vi "16 and 4 pulses TX 1spc.vi"(7 "reset system clock":bool, 8 "referenses":T5={"clock x2"="IO Socket\\Data Clock 2x", "Memory In"="pulse on memory", "Memory In 2"="pulse on memory", "Memory In 3"="pulse on memory", "Memory In 4"="pulse on memory"}, 9 "IQ_run":bool=TRUE, 10 "PDW input Valid":bool, 11 "array PDW":u64[](array[numeric])=[0, 0, 0, 0]) -> (0 "debug mode":T3 {"Cluster"."frequency shift" format="%#_12f"}, 1 "pulse TX status":T6, 2 "output valid":bool, 3 "IQ out":T4, 4 "ready for input":bool)   [LabVIEW 2021]
uses:
  <instrlib>/_niInstr/DSP/v1/Shared/Public/IQ Data.ctl
  pulse_tx_vis/pdw.ctl
  pulse_tx_vis/CTL/mode_type.ctl
  <instrlib>/_niInstr/Basic Elements/v1/FPGA/Private/Count Up U64.vi
  <instrlib>/_niInstr/Basic Elements/v1/FPGA/Private/Count Up U32.vi
  <instrlib>/_niInstr/Basic Elements/v1/FPGA/niInstr Basic Elements v1 FPGA.lvlib
  <instrlib>/_niInstr/DSP/v1/Shared/niInstr DSP v1 Shared.lvlib
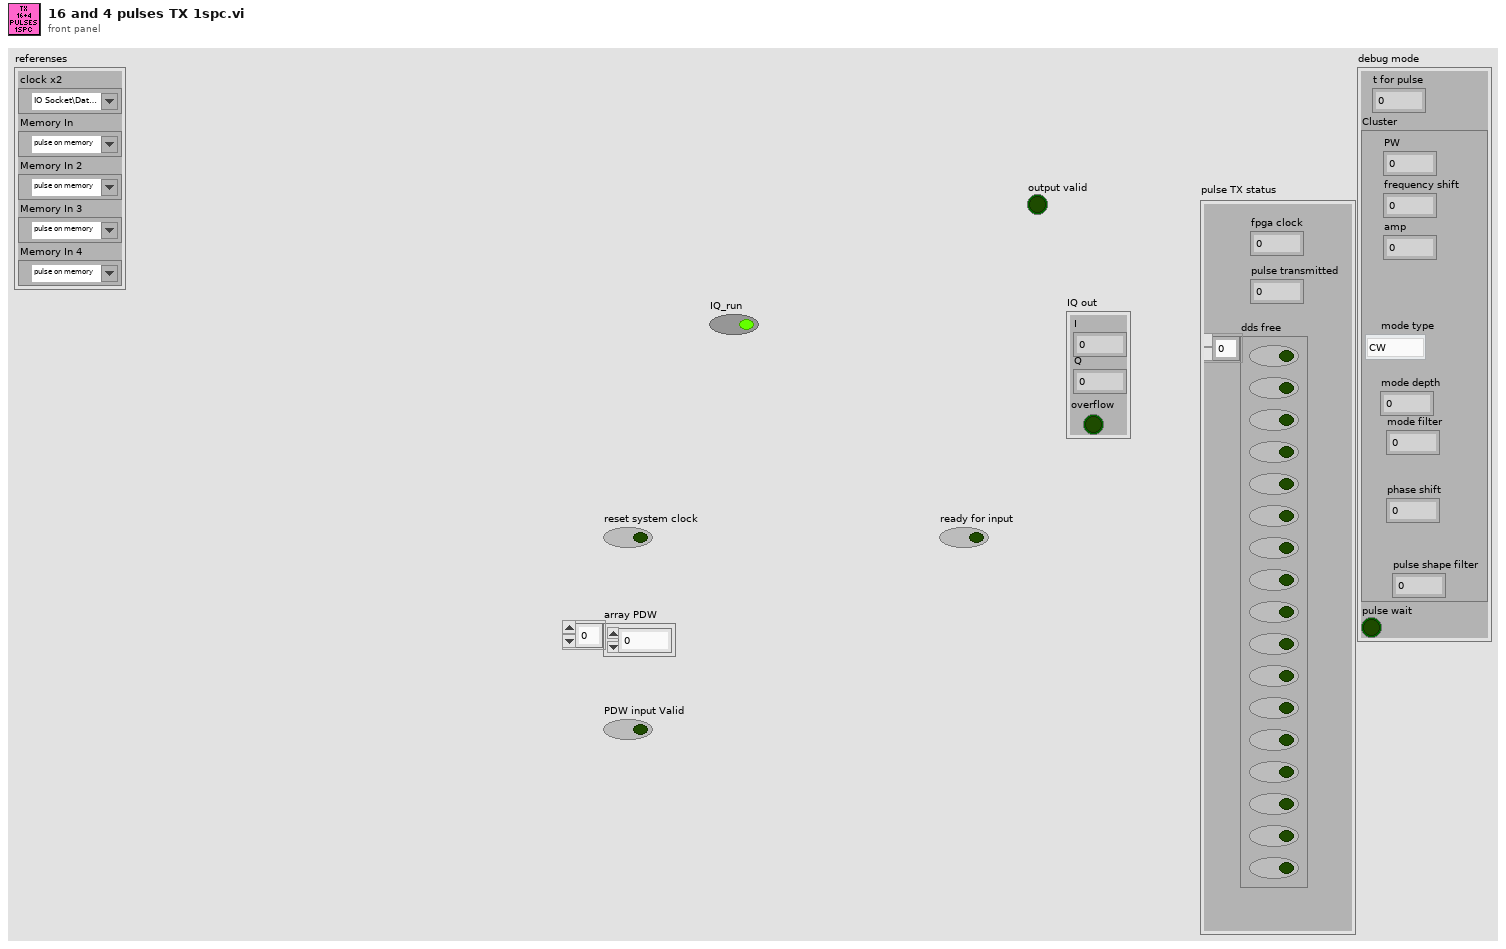
[diagram p1: front panel]
types:
  T1 = typedef "pdw.ctl" = cluster{"PW":u32, "frequency shift":fxp<+/-,48,0>, "amp":fxp<+/-,18,1>, "mode type":T2, "mode depth":u32, "mode filter":u8, "phase shift":fxp<+/-,16,1>, "pulse shape filter":u8}
  T2 = typedef "mode_type.ctl" = enum8{"CW", "from memory 1", "NC - cw", "LFM", "BPSK", "QPSK"}
  T3 = cluster{"t for pulse":u64, "Cluster":T1, "pulse wait":bool}
  T4 = typedef "niInstr DSP v1 Shared.lvlib/IQ Data.ctl" = cluster{"I":fxp<+/-,18,1>, "Q":fxp<+/-,18,1>, "overflow":bool}
  T5 = cluster{"clock x2":refnum<k21>, "Memory In":refnum<k21>, "Memory In 2":refnum<k21>, "Memory In 3":refnum<k21>, "Memory In 4":refnum<k21>}
  T6 = cluster{"fpga clock":u64, "pulse transmitted":u32, "dds free":bool[]}
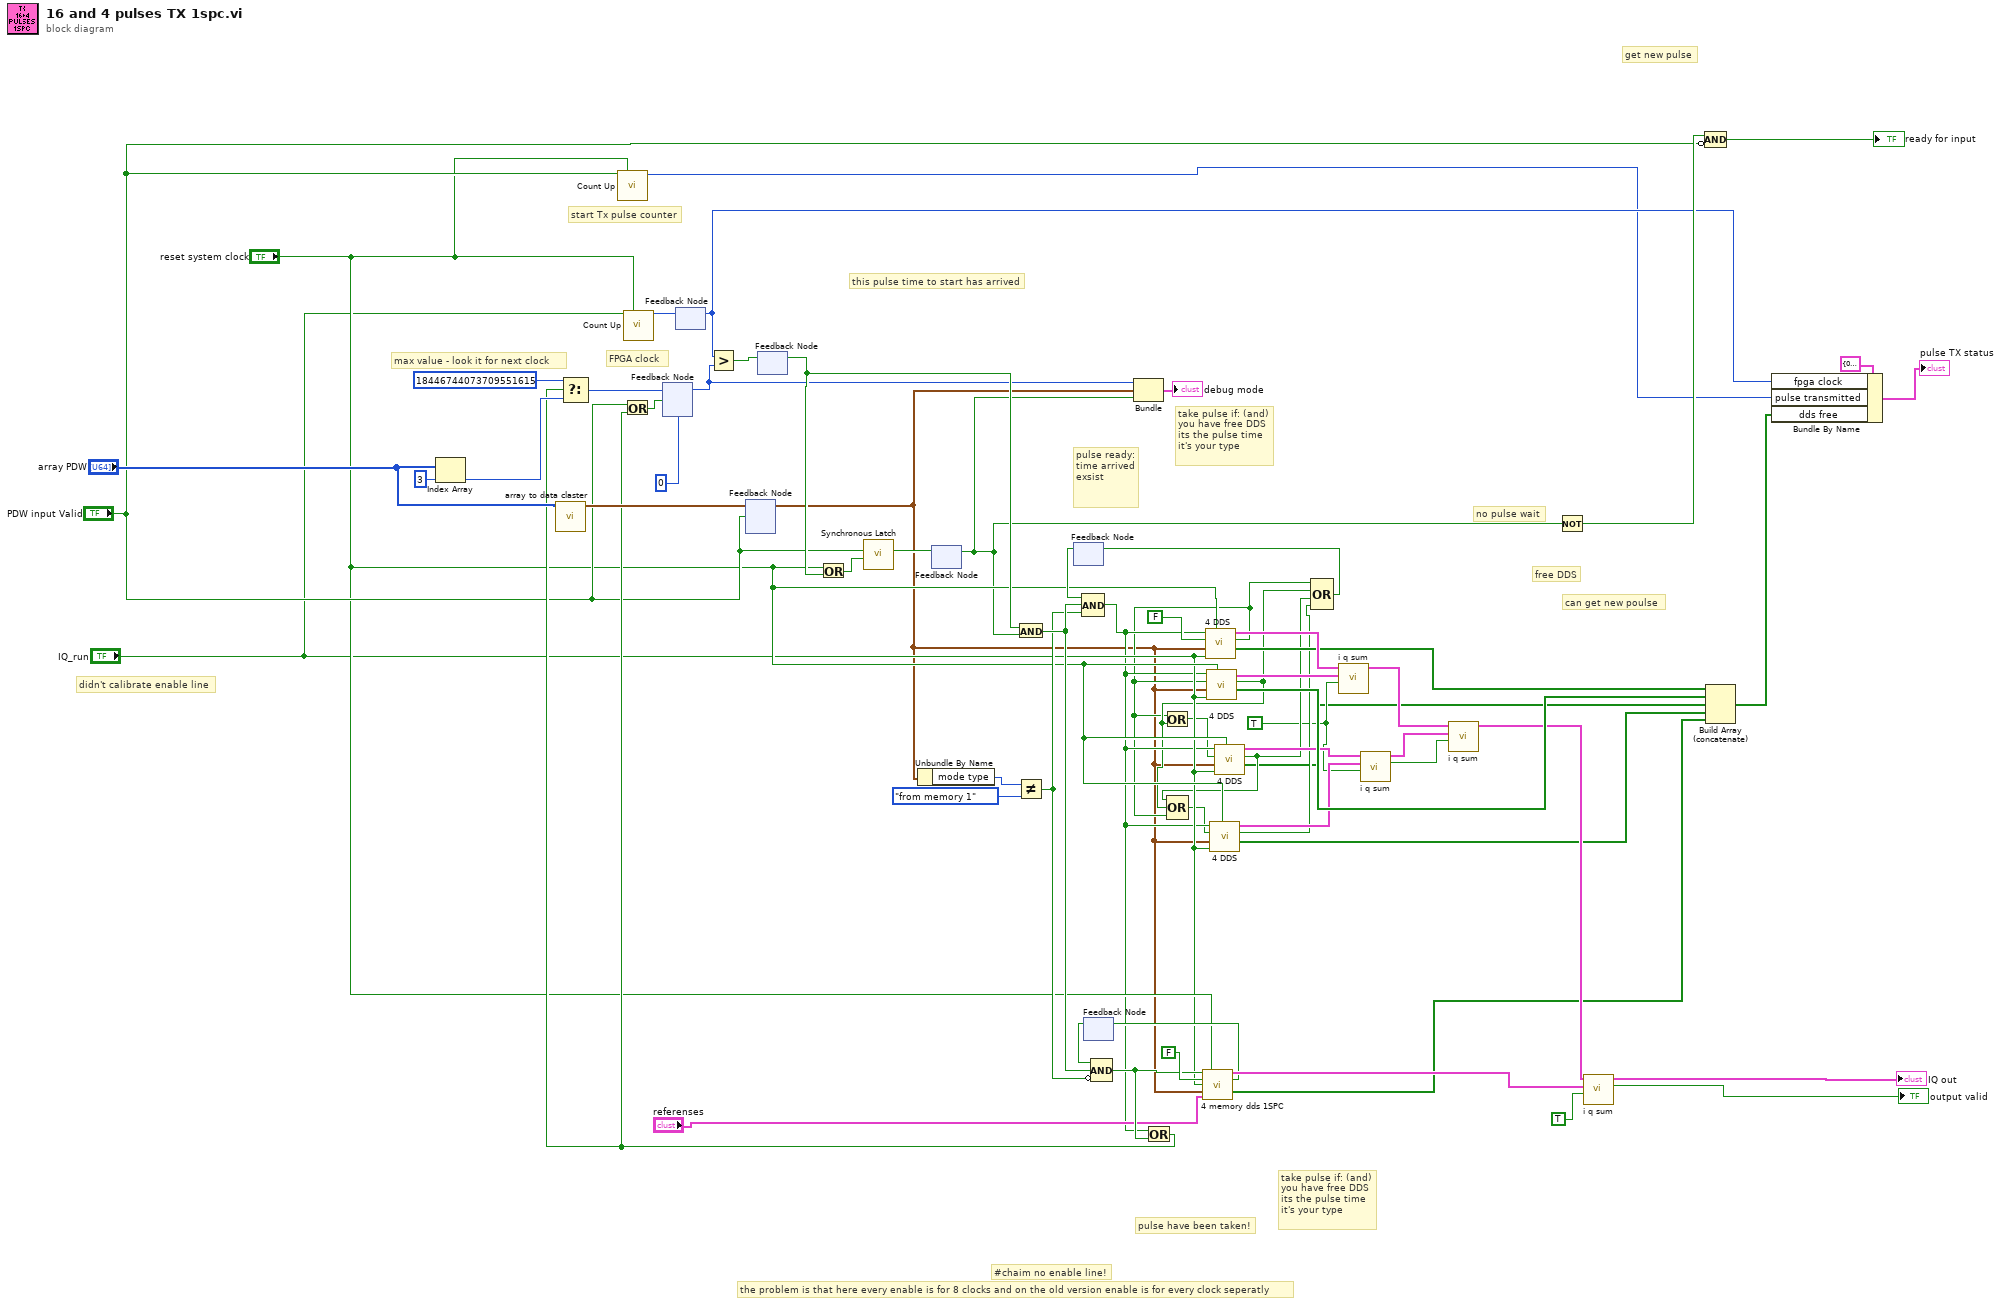
[diagram p0: block diagram]
diagram:
  w12 = TRUE ("input valid")
  # "didn't calibrate enable line"
  # "pulse ready:\ntime arrived\nexsist"
  # "take pulse if: (and)\nyou have free DDS\nits the pulse time\nit's your type"
  # "take pulse if: (and)\nyou have free DDS\nits the pulse time\nit's your type"
  # "pulse have been taken!"
  # "the problem is that here every enable is for 8 clocks and on the old version enable is for every clock seperatly"
  # "#chaim no enable line!"
  # "start Tx pulse counter"
  # "FPGA clock"
  # "this pulse time to start has arrived"
  # "max value - look it for next clock"
  # "get new pulse"
  # "can get new poulse"
  # "no pulse wait"
  # "free DDS"
  n1 = Index Array(array="array PDW", index=3) -> (element=w62:u64)
  n2 = call "array to data claster.vi"("Array"="array PDW") -> ("Cluster"=w46:T1)  [unwired: 10 in]
  n3 = call-poly <instrlib>:"Count Up.vi"("increment"="PDW input Valid", "reset"="reset system clock") -> ("count out"=w50:u32)  [unwired: 13 in]
  n4 = call-poly <instrlib>:"Count Up.vi"("increment"="IQ_run", "reset"="reset system clock") -> ("count out"=w60:u64)  [unwired: 13 in]
  n5 = feedback #1(u64 0 ("U64")) -> (w3:u64)
  n6 = feedback #2() -> (w51:u64)  [unwired: 1 in]
  n7 = feedback-in #2(w60) -> ()
  n8 = Greater?(x=w51, y=w3) -> (0:w65:bool)
  n9 = feedback #3() -> (w4:T1)  [unwired: 1 in]
  n10 = feedback-in #3(w46, "PDW input Valid") -> ()
  n11 = feedback #4() -> (w27:bool)  [unwired: 1 in]
  n12 = feedback-in #4(w65) -> ()
  n13 = Or(x="reset system clock", y=w27) -> (x .or. y?=w28:bool)
  n14 = call <instrlib>:"Synchronous Latch.vi"("clear"=w28, "set"="PDW input Valid") -> ("out"=w25:bool)  [unwired: 9 in]
  n15 = Unbundle By Name(w4) -> ("mode type"=w48:T2)
  n16 = feedback #5() -> (w2:bool)  [unwired: 1 in]
  n17 = feedback-in #5(w25) -> ()
  n18 = And(x=w27, y=w2) -> (x .and. y?=w44:bool)
  n19 = Not Equal?(x=w48, y=mode_type."from memory 1") -> (x != y?=w43:bool)
  n20 = feedback #6() -> (w34:bool)  [unwired: 1 in]
  n21 = Compound Arithmetic op=AND(w34, w44, w43) -> (w19:bool)
  n22 = feedback #7() -> (w38:bool)  [unwired: 1 in]
  n23 = Compound Arithmetic op=AND(w38, w44, invert w43) -> (w37:bool)
  n24 = Bundle("U64"=w3, "Cluster"=w4, "out"=w2) -> (→"debug mode":cluster{"U64":u64, "Cluster":T1, "out":bool})  [unwired: 1 in]
  n25 = Or(x=w19, y=w37) -> (x .or. y?=w36:bool)
  n26 = Select(t=u64 18446744073709551615, s=w36, f=w62) -> (s? t:f=w57:u64)
  n27 = Or(x="PDW input Valid", y=w36) -> (x .or. y?=w58:bool)
  n28 = feedback-in #1(w57, w58) -> ()
  n29 = call "4 memory dds 1SPC.vi"("new PDW in"=w37, "stop this pulse"="reset system clock", "free DDS before me?"=FALSE, "run"="IQ_run", "pdw in"=w4, "referenses"="referenses") -> ("output cluster"=w40:T4, "have free DDS"=w39:bool, "state of every DDS"=w7:bool[])  [unwired: 6 in, 1 out]
  n30 = feedback-in #7(w39) -> ()
  n31 = call "4 DDS.vi"("clear DDS"="reset system clock", "input valid"="IQ_run", "pdw in"=w4, "free DDS before me?"=FALSE, "new PDW in"=w19) -> ("state of every DDS"=w30:bool[], "have free DDS"=w15:bool, "IQ out"=w33:T4)  [unwired: 3 in, 1 out]
  n32 = call "4 DDS.vi"("clear DDS"="reset system clock", "input valid"="IQ_run", "pdw in"=w4, "free DDS before me?"=w15, "new PDW in"=w19) -> ("state of every DDS"=w29:bool[], "have free DDS"=w16:bool, "IQ out"=w32:T4)  [unwired: 3 in, 1 out]
  n33 = Or(x=w15, y=w16) -> (x .or. y?=w18:bool)
  n34 = call "4 DDS.vi"("clear DDS"="reset system clock", "input valid"="IQ_run", "pdw in"=w4, "free DDS before me?"=w18, "new PDW in"=w19) -> ("state of every DDS"=w5:bool[], "have free DDS"=w13:bool, "IQ out"=w23:T4)  [unwired: 3 in, 1 out]
  n35 = Compound Arithmetic op=OR(w13, w16, w15) -> (w17:bool)
  n36 = call "4 DDS.vi"("clear DDS"="reset system clock", "input valid"="IQ_run", "pdw in"=w4, "free DDS before me?"=w17, "new PDW in"=w19) -> ("state of every DDS"=w6:bool[], "have free DDS"=w14:bool, "IQ out"=w22:T4)  [unwired: 3 in, 1 out]
  n37 = Compound Arithmetic op=OR(w15, w16, w13, w14) -> (w31:bool)
  n38 = feedback-in #6(w31) -> ()
  n39 = call "i q sum.vi"("input valid"=w12, 10:"data in"=w32, 11:"data in"=w33) -> ("output cluster"=w11:T4)  [unwired: 7 in, 1 out]
  n40 = call "i q sum.vi"("input valid"=w12, 10:"data in"=w22, 11:"data in"=w23) -> ("output valid"=w9:bool, "output cluster"=w10:T4)  [unwired: 7 in]
  n41 = call "i q sum.vi"("input valid"=w9, 10:"data in"=w10, 11:"data in"=w11) -> ("output cluster"=w8:T4)  [unwired: 7 in, 1 out]
  n42 = Not(x=w2) -> (.not. x?=w54:bool)
  n43 = call "i q sum.vi"("input valid"=TRUE, 10:"data in"=w40, 11:"data in"=w8) -> ("output valid"=→"output valid":bool, "output cluster"=→"IQ out":T4)  [unwired: 7 in]
  n44 = Compound Arithmetic op=AND(w54, invert "PDW input Valid") -> (→"ready for input":bool)
  n45 = Build Array (concatenate)(w30, w29, w5, w6, w7) -> (w49:bool[])
  n46 = Bundle By Name(cluster=T6 {"fpga clock"=0, "pulse transmitted"=0, "dds free"=[FALSE, FALSE, FALSE, FALSE, FALSE, FALSE, FALSE, FALSE, FALSE, FALSE, FALSE, FALSE, FALSE, FALSE, FALSE, FALSE, FALSE, FALSE, FALSE, FALSE]} ("pulse TX status"), "fpga clock"=w51, "pulse transmitted"=w50, "dds free"=w49) -> (→"pulse TX status":T6)
